vi "Format 1D.vi"(1 "X 1D Array":dbl[](array[numeric]), 2 "X  Array name":string) -> (0 "String":string)   [LabVIEW 2016, in "LVtoITX.lvclass"]
uses:
  LVtoITX.lvclass
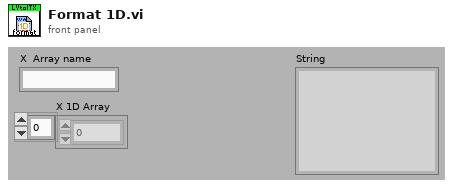
[diagram p1: front panel]
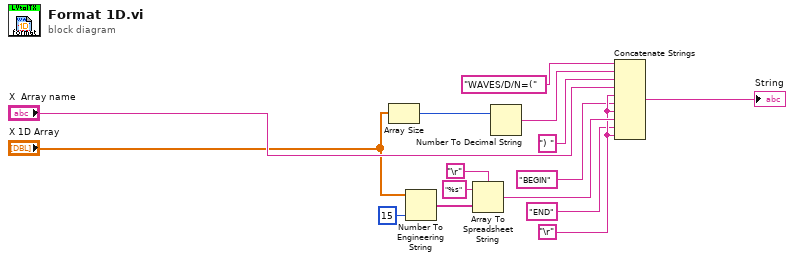
[diagram p0: block diagram]
diagram:
  w9 = "\r"
  n1 = Array Size(array="X 1D Array") -> (size(s)=w4:i32)
  n2 = Number To Engineering String(2:i16 15 ("precision (6)"), 4:"X 1D Array") -> (0:w2:string[])  [unwired: 2 out]
  n3 = Array To Spreadsheet String(delimiter (Tab)="\r", array=w2, 3:"%s" ("format string")) -> (spreadsheet string=w10:string)
  n4 = Number To Decimal String(number=w4) -> (decimal integer string=w12:string)  [unwired: 1 out]
  n5 = Concatenate Strings("WAVES/D/N=(", w12, ") ", "X  Array name", w9, "BEGIN", w9, w10, "END", w9) -> (→"String":string)
